vi "Tree_Duplicate Tree.vi"(6 "Number of Child Columns to Replicate":i32=-1 min=-1, 8 "error in (no error)":errorcluster, 10 "New Tree":refnum<vi>, 11 "Old Tree":refnum<vi>) -> (0 "error out":errorcluster, 2 "dup New Tree":refnum<vi>, 3 "dup Old Tree":refnum<vi>)   [LabVIEW 2020]
doc: "This VI takes a reference to a populated tree control (Old Tree) and an empty tree control (New Tree). The VI will then replicate the contents of Old Tree within New Tree. Optionally, you can specify how many child columns you wish to replicate. The default value (-1) indicates that you want to duplicate all visible columns in Old Tree."
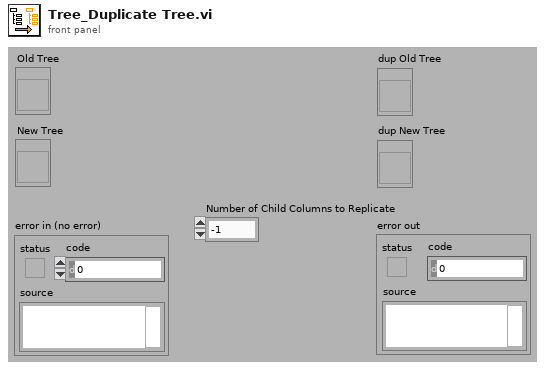
[diagram p1: front panel]
types:
  T1 = cluster{"Cell String":string, string[], string, "Indent Level":i32, "Child-Only?":bool, "Glyph":i32}
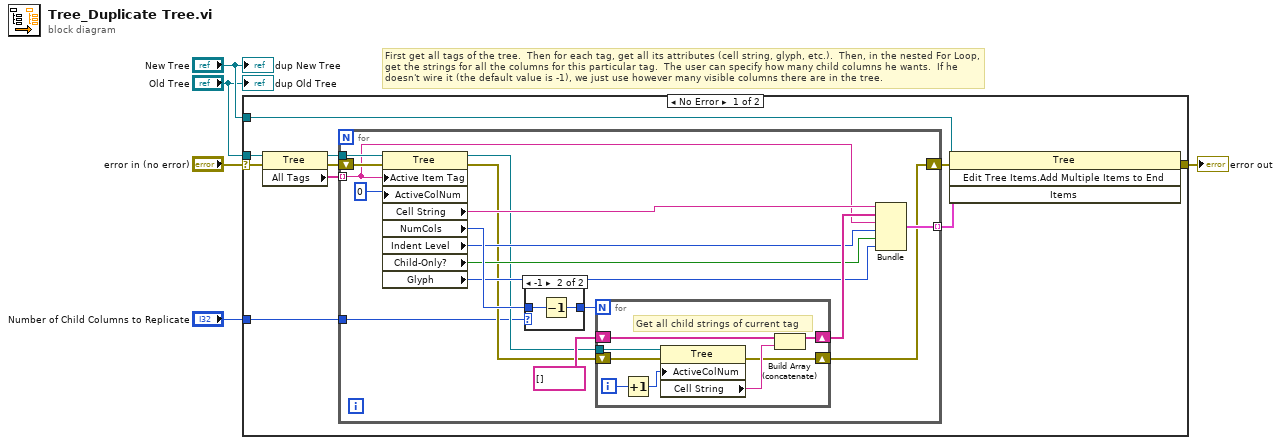
[diagram p0: block diagram]
diagram:
  # "First get all tags of the tree.  Then for each tag, get all its attributes (cell string, glyph, etc.).  Then, in the nested For Loop, get the strings for all the columns for this particular tag.  The user can specify how many child columns he wants.  If he doesn't wire it (the default value is -1), we just use however many visible columns there are in the tree."
  n1 = case shown="No Error" "error in (no error)" {
    selector: "error in (no error)" -> [w7 w44]
    tunnel: [w11 w44] -> w5
    tunnel: "New Tree" -> [w9 _]
    tunnel: "Old Tree" -> [w8 _]
    tunnel: "Number of Child Columns to Replicate" -> [w6 _]
    frame No Error {
      n2 = property on="Property Node" class="Tree"(reference=w8, error in=w7) -> (reference out=w14:refnum<vi>, error out=w13:errorcluster, "All Tags"=w15:string[])
      n3 = for {
        tunnel: w15 -> [w24] mode=indexing
        tunnel: w14 -> [w32]
        tunnel: [w20] -> w12 mode=indexing
        shift-right: [w17] -> w10
        shift-left: w13 -> [w31]
        tunnel: w6 -> [w16]
        n4 = property on="Property Node" class="Tree"(reference=w32, error in=w31, "Active Item Tag"=w24, "ActiveColNum"=0 ("Active Cell:Active Column Number")) -> (reference out=w19:refnum<vi>, error out=w18:errorcluster, "Cell String"=w29:string, "NumCols"=w28:u32, "Indent Level"=w23:i32, "Child-Only?"=w22:bool, "Glyph"=w21:i32)
        n5 = case shown="-1" w16 {
          selector: w16 -> [w33 _]
          tunnel: w28 -> [_ w35]
          tunnel: [w33 w34] -> w27
          frame Default {
          }
          frame -1 {
            n6 = Decrement(x=w35) -> (x-1=w34:u32)
          }
        }
        n7 = for {
          N: w27 -> [_]
          shift-right: [w41] -> w25
          shift-left: string[] [] -> [w42]
          tunnel: w19 -> [w39]
          shift-right: [w36] -> w17
          shift-left: w18 -> [w37]
          i -> [w43]
          # "Get all child strings of current tag"
          n8 = Increment(x=w43) -> (x+1=w38:i32)
          n9 = property on="Property Node" class="Tree"(reference=w39, error in=w37, "ActiveColNum"=w38) -> (error out=w36:errorcluster, "Cell String"=w40:string)  [unwired: 1 out]
          n10 = Build Array (concatenate)(w42, w40) -> (w41:string[])
        }
        n11 = Bundle("Cell String"=w29, w25, w24, "Indent Level"=w23, "Child-Only?"=w22, "Glyph"=w21) -> (w20:T1)  [unwired: 1 in]
      }
      n12 = invoke on="Invoke Node" class="Tree" method="Edit Tree Items.Add Multiple Items to End"(reference=w9, error in=w10, "Items"=w12) -> (error out=w11:errorcluster)  [unwired: 1 in, 3 out]
    }
    frame Error {
    }
  }
  "error out" <- w5
  "dup Old Tree" <- "Old Tree"
  "dup New Tree" <- "New Tree"
